vi "DeleteScript-TestManager.vi"() -> (0 "error out":errorcluster, 3 "Tags after deletion":string[](array[string]))   [LabVIEW 2018]
panel:
  in  "error in (no error)":errorcluster
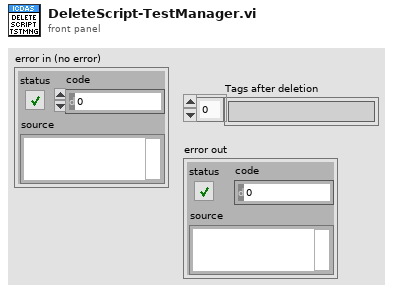
[diagram p1: front panel]
types:
  T1 = typedef "cntlRefs.ctl" = cluster{"rngFGen":refnum<vi>, "rngDigitizer":refnum<vi>, "btnHide":refnum<vi>, "rngInst":refnum<vi>, "Instrument Modules":refnum<vi>, "RelativePathToINIFiles ":refnum<vi>, "PluginTree":refnum<vi>, "TestListboxRef":refnum<vi>, "path.tstFile":refnum<vi>, "cmbxRunningModules":refnum<vi>, "TestDataSubPanel":refnum<vi>, "TestDataCaption":refnum<vi>, "btnPopInOut":refnum<vi>, "PluginMgrQ":refnum<queue>, "TestMgrQ":refnum<queue>, "TestMgrSubPanel":refnum<vi>, "PluginMgrSubPanel":refnum<vi>, "PwrReqHandle":u32, "btnStopOneTest":refnum<vi>, "pathUserfiles":refnum<vi>, "PluginTreeCaption":refnum<vi>, "MainVIRef":refnum<vi>}
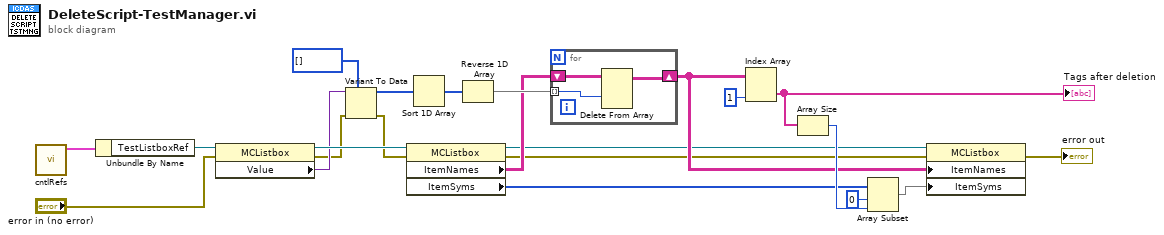
[diagram p0: block diagram]
diagram:
  n1 = call "cntlRefs.vi"() -> ("cntlRefs"=w8:T1)  [unwired: 10 in, 1 out]
  n2 = Unbundle By Name(w8) -> ("TestListboxRef"=w12:refnum<vi>)
  n3 = property class="MCListbox"(reference=w12, error in="error in (no error)") -> (reference out=w7:refnum<vi>, error out=w3:errorcluster, "Value"=w6:variant)
  n4 = Variant To Data(error in=w3, type=i32[] [] ("Value"), Variant=w6) -> (data=w4:i32[], error out=w2:errorcluster)
  n5 = property class="MCListbox"(reference=w7, error in=w2) -> (reference out=w10:refnum<vi>, error out=w11:errorcluster, "ItemNames"=w14:string[][], "ItemSyms"=w19:i32[])
  n6 = Sort 1D Array(array=w4) -> (sorted array=w13:i32[])
  n7 = Reverse 1D Array(array=w13) -> (reversed array=w15:i32[])
  n8 = for {
    shift-right: [w23] -> w17
    shift-left: w14 -> [w25]
    tunnel: w15 -> [w24] mode=indexing
    n9 = Delete From Array(array=w25, index (row)=w24) -> (array with subset deleted=w23:string[][])  [unwired: 2 in, 1 out]
  }
  n10 = Index Array(array=w17, index (col)=1 ("disabled index (col)")) -> (element=w18:string[])  [unwired: 1 in]
  "Tags after deletion" <- w18
  n11 = Array Size(array=w18) -> (size(s)=w20:i32)
  n12 = Array Subset(array=w19, index=0, length=w20) -> (w22:i32[])
  n13 = property class="MCListbox"(reference=w10, error in=w11, "ItemNames"=w17, "ItemSyms"=w22) -> (error out=→"error out":errorcluster)  [unwired: 1 out]
